vi "decide_where_to_move--Warndorff's rule.vi"(2 "tour_in_progress":T1[](array[typedef]), 3 "chessboard":T2[][](array[typedef])) -> (0 "square_to_move_forward_to":T1, 1 "action":T4)   [LabVIEW 2020, in "core.lvlib"]
uses:
  core.lvlib
  action.ctl
  core_data/chessboard_index.ctl
  core_data/chess_square.ctl
  core_data/neighbour_square.ctl
  pause (global variable).vi
  core_data/core_data.lvlib
panel:
  # "Development\ncontrols/indicators useful for development and testing, but which are not outputs of the VI"
  # "Input\nInputs to the VI"
  # "Output\nOutputs of the VI"
  # "Description\n\nBlank VI with error handling case. \n\nSummarize the use of this VI in this space."
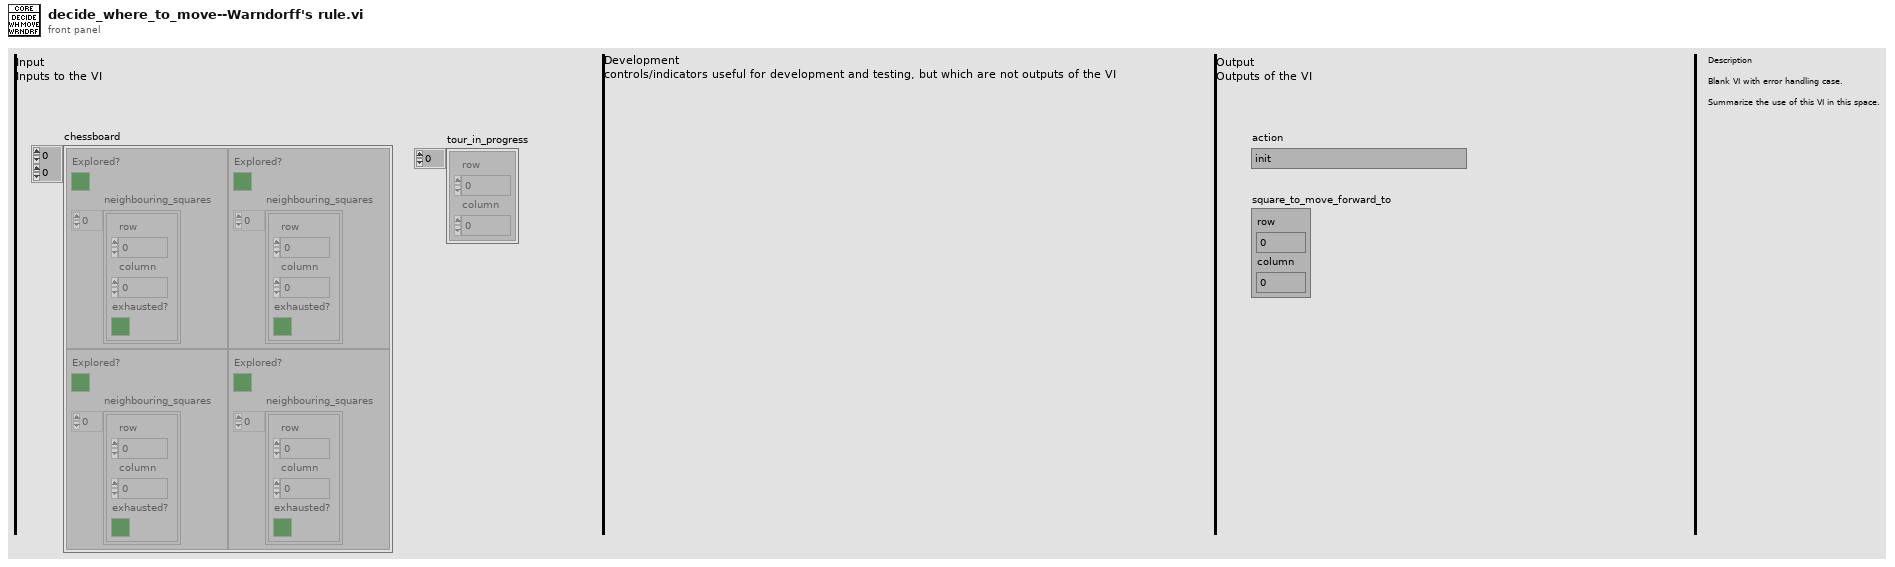
[diagram p1: front panel]
types:
  T1 = typedef "core.lvlib/core_data.lvlib/chessboard_index.ctl" = cluster{"row":u8, "column":u8}
  T2 = typedef "core.lvlib/core_data.lvlib/chess_square.ctl" = cluster{"Explored?":bool, "neighbouring_squares":T3[]}
  T3 = typedef "core.lvlib/core_data.lvlib/neighbour_square.ctl" = cluster{"row":u8, "column":u8, "exhausted?":bool}
  T4 = typedef "core.lvlib/action.ctl" = enum16{"init", "move_forward", "move_backward", "complete_tour", "exit", "be idle (do nothing)"}
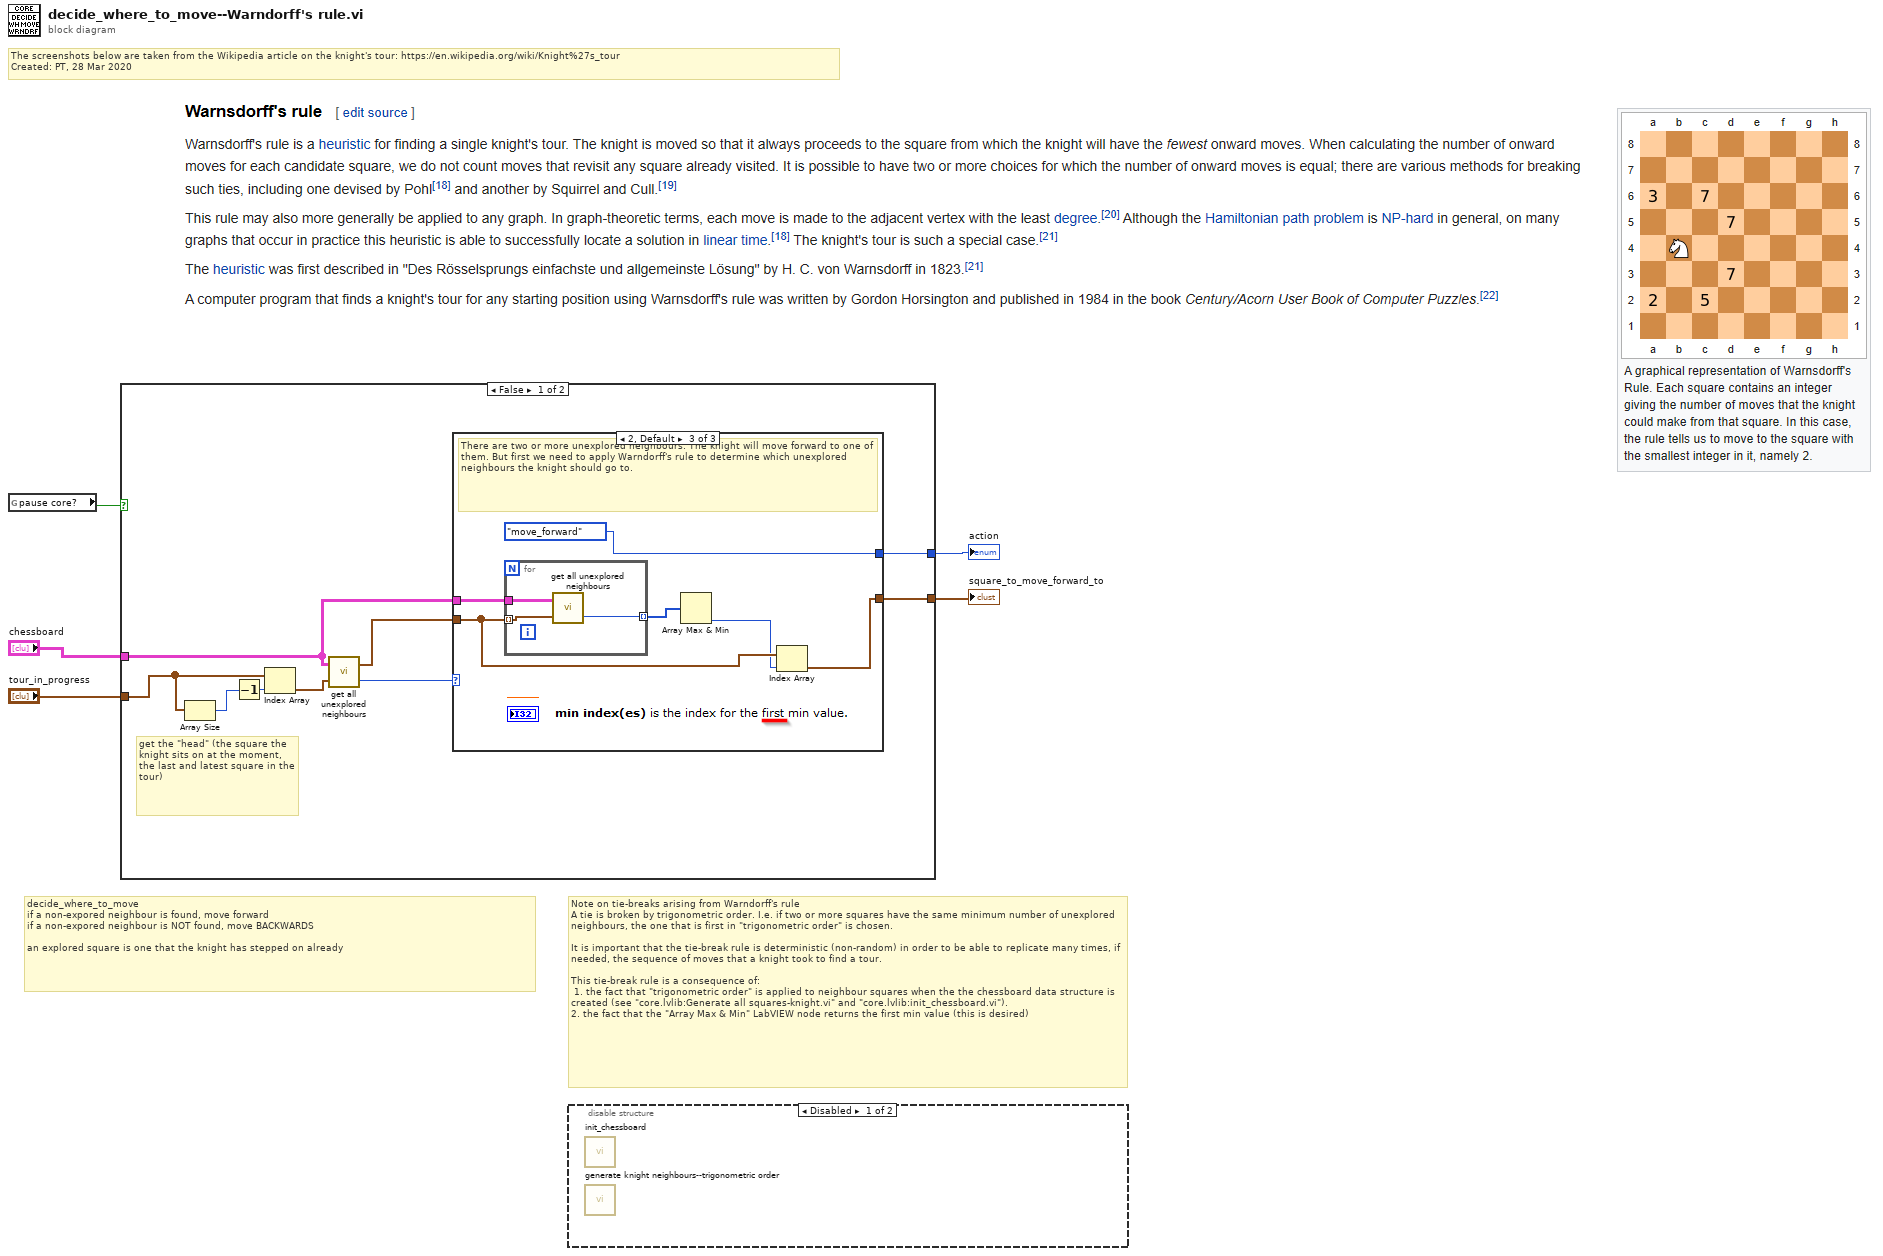
[diagram p0: block diagram]
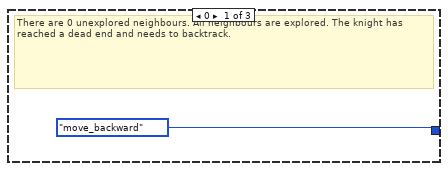
[diagram p3: hidden frame]
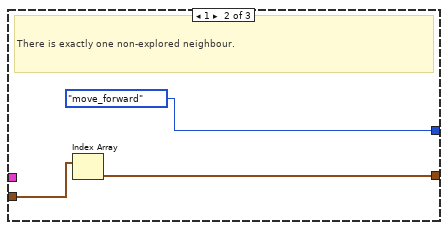
[diagram p4: hidden frame]
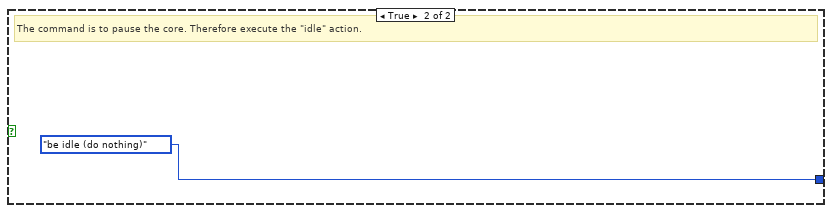
[diagram p5: hidden frame]
diagram:
  # "Note on tie-breaks arising from Warndorff's rule\nA tie is broken by trigonometric order. I.e. if two or more squares have the same minimum number of unexplored neighbours, the one that is first in \"trigonometric order\" is chosen.\n\nIt is important that the tie-break rule is deterministic (non-random) in order to be able to replicate many times, if needed, the sequence of moves that a knight took to find a tour.\n\nThis tie-break rule is a consequence of:\n 1. the fact that \"trigonometric order\" is applied to neighbour squares when the the chessboard data structure is created (see \"core.lvlib:Generate all squares-knight.vi\" and \"core.lvlib:init_chessboard.vi\").\n2. the fact that the \"Array Max & Min\" LabVIEW node returns the first min value (this is desired)"
  # "decide_where_to_move\nif a non-expored neighbour is found, move forward\nif a non-expored neighbour is NOT found, move BACKWARDS\n\nan explored square is one that the knight has stepped on already"
  # "The screenshots below are taken from the Wikipedia article on the knight's tour: https://en.wikipedia.org/wiki/Knight%27s_tour \nCreated: PT, 28 Mar 2020"
  n1 = global read "pause (global variable).vi" "pause core?"() -> (w4:bool)
  n2 = case shown="False" w4 {
    tunnel: [w14 action."be idle (do nothing)" ("action")] -> w5
    tunnel: "chessboard" -> [w7 _]
    tunnel: "tour_in_progress" -> [w11 _]
    tunnel: [w10 _] -> w1
    frame False {
      # "get the \"head\" (the square the knight sits on at the moment, the last and latest square in the tour)"
      n3 = Array Size(array=w11) -> (size(s)=w12:i32)
      n4 = Decrement(x=w12) -> (x-1=w13:i32)
      n5 = Index Array(array=w11, index=w13) -> (element=w9:T1)
      n6 = call "get all unexplored neighbours.vi"("square (chessboard index)"=w9, "chessboard"=w7) -> ("no. of unexplored neighbours"=w6:i32, "unexplored neighbours"=w8:T1[])
      n7 = case shown="2, Default" w6 {
        tunnel: [action."move_backward" ("action") action."move_forward" ("action") action."move_forward" ("action")] -> w14
        tunnel: w8 -> [_ w17 w21]
        tunnel: [_ w16 w19] -> w10
        tunnel: w7 -> [_ _ w23]
        frame 0 {
          # "There are 0 unexplored neighbours. All neighbours are explored. The knight has reached a dead end and needs to backtrack."
        }
        frame 1 {
          # "There is exactly one non-explored neighbour."
          n8 = Index Array(array=w17) -> (element=w16:T1)  [unwired: 1 in]
        }
        frame 2, Default {
          # "There are two or more unexplored neighbours. The knight will move forward to one of them. But first we need to apply Warndorff's rule to determine which unexplored neighbours the knight should go to."
          n9 = for {
            tunnel: w23 -> [w27]
            tunnel: w21 -> [w26] mode=indexing
            tunnel: [w25] -> w22 mode=indexing
            n10 = call "get all unexplored neighbours.vi"("square (chessboard index)"=w26, "chessboard"=w27) -> ("no. of unexplored neighbours"=w25:i32)  [unwired: 1 out]
          }
          n11 = Array Max & Min(array=w22) -> (min index (indices)=w20:i32)  [unwired: 3 out]
          n12 = Index Array(array=w21, index=w20) -> (element=w19:T1)
        }
      }
    }
    frame True {
      # "The command is to pause the core. Therefore execute the \"idle\" action."
    }
  }
  "action" <- w5
  "square_to_move_forward_to" <- w1
  n13 = disable-structure shown="Disabled" {
    frame Disabled {
      n14 = call "init_chessboard.vi"() -> ()  [unwired: 10 in, 2 out]
      n15 = call "generate knight neighbours--trigonometric order.vi"() -> ()  [unwired: 1 in, 1 out]
    }
    frame Enabled {
    }
  }
